vi "Sync2.vi"(8 "Input Stream":dbl[](array[numeric]), 9 "error in (no error)":errorcluster, 10 "Frame Instruction":T1, 11 "PN sequence order (9)":i32=9) -> (1 "Output Stream":dbl[][](array[numeric]), 2 "error out":errorcluster)   [LabVIEW 2014]
uses:
  <vilib>/addons/Modulation/Digital/General/MT Generate Bits (Galois, PN Order).vi
  <vilib>/addons/Modulation/Digital/Support/Common/Validators/mod_Generate Bits Validate.vi
  <vilib>/addons/Modulation/Analog/support/mod_Set Error Source.vi
  <vilib>/addons/Modulation/Digital/General/subVIs/mod_Generate Bits PN Sequence.vi
  <vilib>/addons/Modulation/niDMT.lvlib
panel:
  out "Message Data":dbl
  out "Numeric 3":i32
  out "Array 3":i32[](array[numeric])
  out "Numeric 2":dbl
  out "Numeric":dbl
  out "Array 2":dbl[](array[numeric])
  out "Array":dbl[](array[numeric])
  out "output bit stream":i8[](array[numeric])
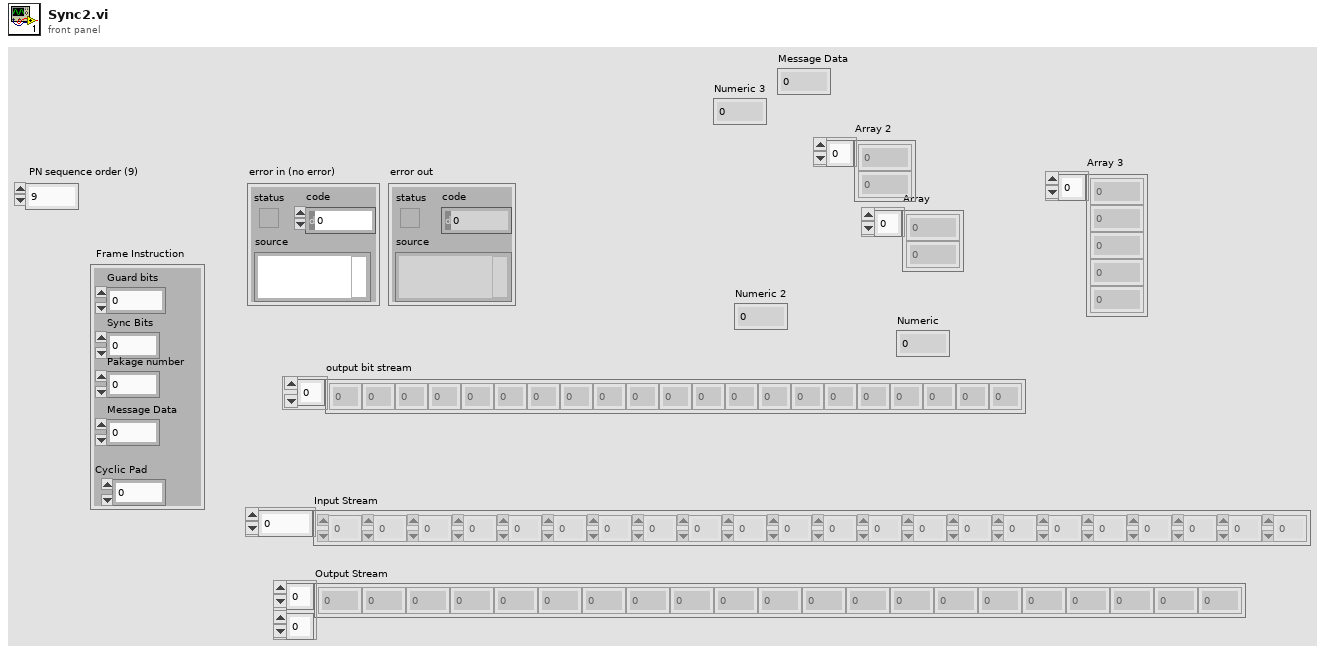
[diagram p1: front panel]
types:
  T1 = cluster{"Guard bits":dbl, "Sync Bits":dbl, "Pakage number":dbl, "Cyclic Pad":dbl, "Message Data":dbl}
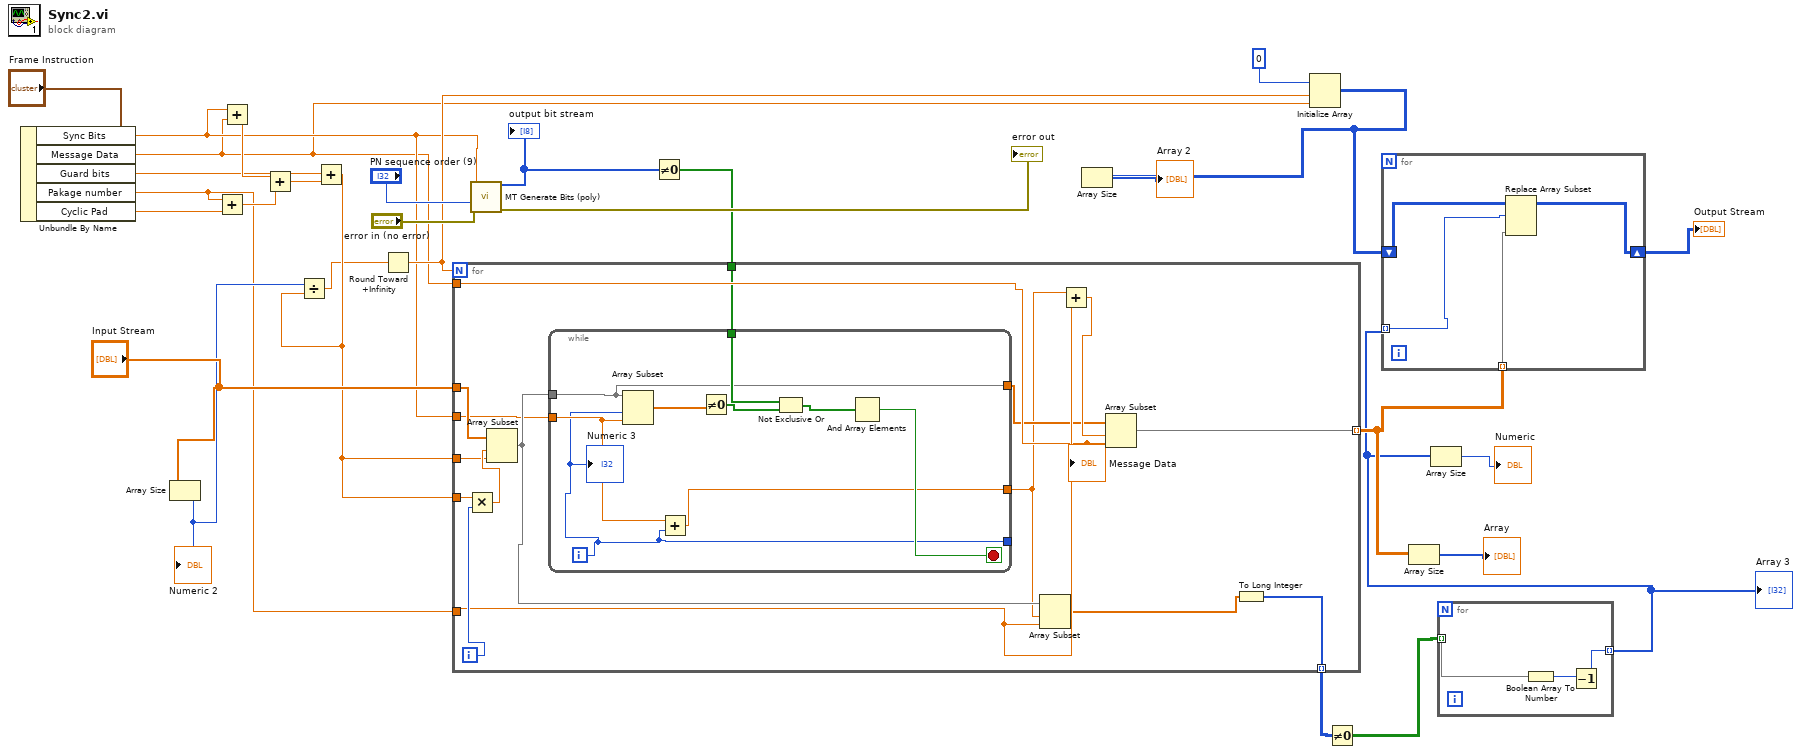
[diagram p0: block diagram]
diagram:
  n1 = Unbundle By Name("Frame Instruction") -> ("Sync Bits"=w3:dbl, "Message Data"=w2:dbl, "Guard bits"=w22:dbl, "Pakage number"=w1:dbl, "Cyclic Pad"=w25:dbl)
  n2 = Array Size(array="Input Stream") -> (size(s)=w14:i32)
  "Numeric 2" <- w14
  n3 = Add(x=w1, y=w25) -> (x+y=w23:dbl)
  n4 = Add(x=w3, y=w2) -> (x+y=w24:dbl)
  n5 = Add(x=w24, y=w23) -> (x+y=w21:dbl)
  n6 = Add(x=w22, y=w21) -> (x+y=w13:dbl)
  n7 = Divide(x=w14, y=w13) -> (x/y=w12:dbl)
  n8 = Round Toward +Infinity(x=w12) -> (ceil(x): smallest int >= x=w11:dbl)
  n9 = call-poly <vilib>:"MT Generate Bits (poly).vi"("total bits (128)"=w3, "PN sequence order (9)"="PN sequence order (9)", "error in (no error)"="error in (no error)") -> ("output bit stream"=w8:i8[], "error out"=→"error out":errorcluster)  [unwired: 10 in, 1 out]
  "output bit stream" <- w8
  n10 = Not Equal To 0?(x=w8) -> (x != 0?=w7:bool[])
  n11 = for {
    N: w11 -> [_]
    tunnel: "Input Stream" -> [w42]
    tunnel: w3 -> [w33]
    tunnel: w2 -> [w40]
    tunnel: w13 -> [w44]
    tunnel: w1 -> [w41]
    tunnel: [w31] -> w18 mode=indexing
    tunnel: w13 -> [w38]
    tunnel: [w36] -> w10 mode=indexing
    tunnel: w7 -> [w35]
    i -> [w45]
    n12 = Multiply(x=w44, y=w45) -> (x*y=w43:dbl)
    n13 = Array Subset(array=w42, index=w43, length=w38) -> (w34:dbl[])
    n14 = while {
      tunnel: w34 -> [w49]
      tunnel: w33 -> [w48]
      tunnel: w35 -> [w53]
      tunnel: [w49] -> w32
      tunnel: [w47] -> w30
      tunnel: [w46] -> _
      i -> [w46]
      stop <- w50 stop-if-true
      n15 = Array Subset(array=w49, index=w46, length=w48) -> (w54:dbl[])
      n16 = Add(x=w48, y=w46) -> (x+y=w47:dbl)
      n17 = Not Equal To 0?(x=w54) -> (x != 0?=w52:bool[])
      n18 = Not Exclusive Or(1:w52, 2:w53) -> (0:w51:bool[])
      n19 = And Array Elements(Boolean array=w51) -> (logical AND=w50:bool)
      "Numeric 3" <- w46
    }
    n20 = Array Subset(array=w34, index=w30, length=w41) -> (w37:dbl[])
    n21 = Add(x=w30, y=w41) -> (x+y=w39:dbl)
    n22 = Array Subset "Array Subset"(array=w32, index=w39, length=w40) -> (w31:dbl[])
    n23 = To Long Integer(number=w37) -> (32bit integer=w36:i32[])
    "Message Data" <- w40
  }
  n24 = Initialize Array(0, w11, w2) -> (w5:i32[][])
  n25 = Array Size(array=w5) -> (size(s)=→"Array 2":i32[])
  n26 = Not Equal To 0?(x=w10) -> (x != 0?=w9:bool[][])
  n27 = Array Size(array=w18) -> (size(s)=→"Array":i32[])
  n28 = for {
    tunnel: w9 -> [w56] mode=indexing
    tunnel: [w55] -> w6 mode=indexing
    n29 = Boolean Array To Number(Boolean array=w56) -> (number=w57:u32)
    n30 = Decrement(x=w57) -> (x-1=w55:u32)
  }
  "Array 3" <- w6
  n31 = for {
    tunnel: w6 -> [w60] mode=indexing
    tunnel: w18 -> [w61] mode=indexing
    shift-right: [w58] -> w4
    shift-left: w5 -> [w59]
    n32 = Replace Array Subset(array=w59, new element=w61, index (row)=w60) -> (w58:i32[][])  [unwired: 1 in]
  }
  "Output Stream" <- w4
  n33 = Array Size(array=w6) -> (size(s)=→"Numeric":i32)
